vi "ReadOscilloscopeDataFile.vi"(4 "iteration number":i32, 6 "Channel Index":i32, 7 "Resolution":string, 8 "error in (no error)":errorcluster, 9 "Channel Names":string[][](array[string]), 10 "TimeVoltageData":dbl[][](array[numeric]), 11 "Oscilloscope Data Path":path) -> (0 "error out":errorcluster)   [LabVIEW 2019]
uses:
  <vilib>/Utility/file.llb/Write Delimited Spreadsheet (string).vi
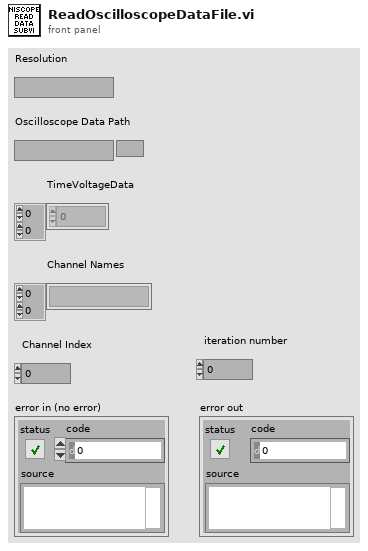
[diagram p1: front panel]
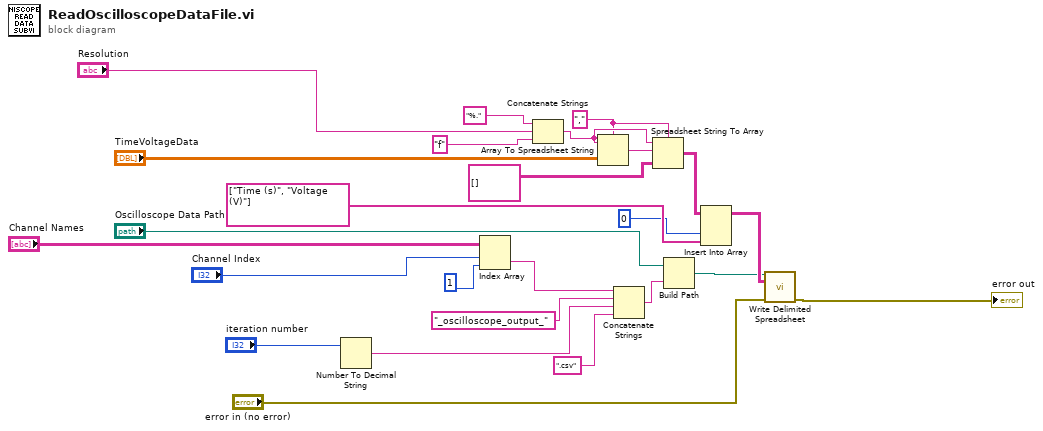
[diagram p0: block diagram]
diagram:
  w10 = "," ("delimiter (Tab)")
  n1 = Number To Decimal String(number="iteration number") -> (decimal integer string=w2:string)  [unwired: 1 in]
  n2 = Index Array(array="Channel Names", index (row)="Channel Index", index (col)=1 ("disabled index (col)")) -> (element=w19:string)
  n3 = Concatenate Strings("%." ("string"), "Resolution", "f" ("string")) -> (w14:string)
  n4 = Array To Spreadsheet String(delimiter (Tab)=w10, array="TimeVoltageData", 3:w14) -> (spreadsheet string=w11:string)
  n5 = Concatenate Strings(w19, "_oscilloscope_output_", w2, ".csv" ("string")) -> (w22:string)
  n6 = Spreadsheet String To Array(delimiter (Tab)=w10, format string=w14, spreadsheet string=w11, array type (2D Dbl)=string[][] []) -> (array=w13:string[][])
  n7 = Build Path(base path="Oscilloscope Data Path", name or relative path=w22) -> (appended path=w8:path)
  n8 = Insert Into Array(array=w13, index (col)=0 ("disabled index (col)"), new element=string[] ["Time (s)", "Voltage (V)"]) -> (w16:string[][])  [unwired: 1 in]
  n9 = call-poly <vilib>:"Write Delimited Spreadsheet.vi"("file path (dialog if empty)"=w8, "2D data"=w16, "error in (no error)"="error in (no error)") -> ("error out"=→"error out":errorcluster)  [unwired: 11 in, 1 out]
